vi "Init.vi"(8 "error in (no error)":errorcluster, 10 "Node Reg":refnum<k20>, 11 "Loop in":refnum<class "Loop.lvclass">) -> (0 "error out":errorcluster, 3 "Loop out":refnum<class "Loop.lvclass">)   [LabVIEW 2025, in "Loop.lvclass"]
uses:
  Loop.lvclass
  Controls/Shift Register.ctl
  Controls/Terminal.ctl
  Structure.lvclass
  <vilib>/xml/NI_XML.lvlib
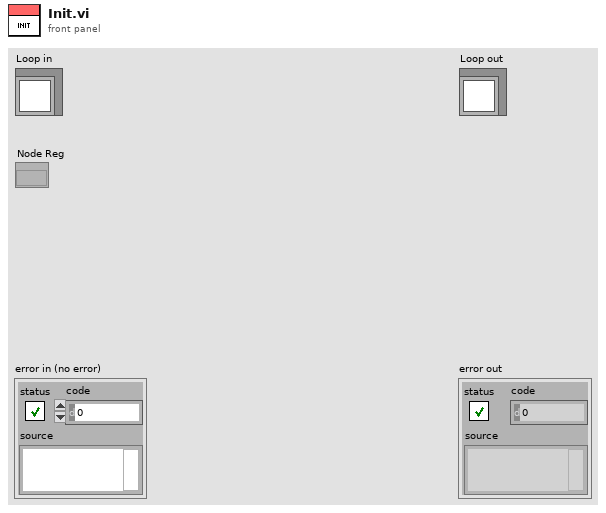
[diagram p1: front panel]
types:
  T1 = typedef "Shift Register.ctl" = cluster{"name":string, "LH Ext":T2, "LH Int":T2, "RH Int":T2, "RH Ext":T2, "Y pos":u32}
  T2 = typedef "Terminal.ctl" = cluster{"id":string, "name":string, "terminal":refnum<vi>}
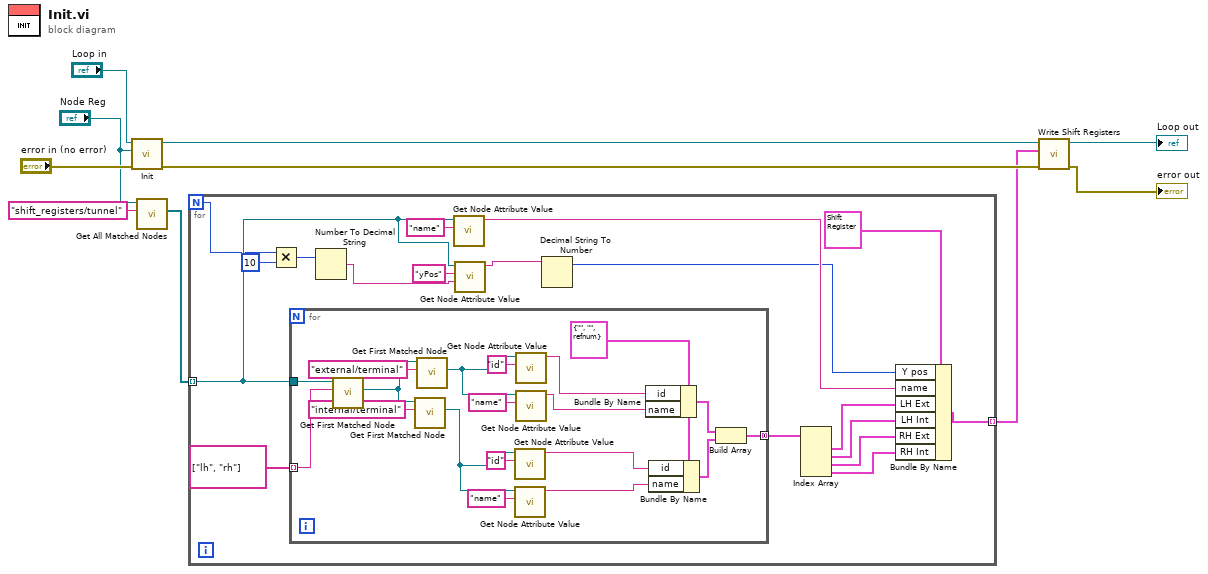
[diagram p0: block diagram]
diagram:
  n1 = call-parent "Init.vi"("error in (no error)"="error in (no error)", "Node Reg"="Node Reg", "Structure in"="Loop in") -> ("error out"=w8:errorcluster, "Structure out"=w7:refnum<class "Loop.lvclass">)  [unwired: 7 in]
  n2 = call <vilib>:"Get All Matched Nodes.vi"("XPath expression"="shift_registers/tunnel", "node in"="Node Reg") -> ("node result array"=w2:refnum<k20>[])  [unwired: 7 in, 2 out]
  n3 = for {
    N -> [w14]
    tunnel: w2 -> [w18] mode=indexing
    tunnel: [w19] -> w1 mode=indexing
    n4 = Multiply(x=w14, y=10) -> (x*y=w12:i32)
    n5 = for {
      tunnel: w18 -> [w47]
      tunnel: string[] ["lh", "rh"] -> [w46] mode=indexing
      tunnel: [w29] -> w27 mode=concatenating
      w34 = T2 {"id"="", "name"="", "terminal"=refnum} ("Terminal")
      n6 = call <vilib>:"Get First Matched Node.vi"("XPath expression"=w46, "node in"=w47) -> ("node result"=w45:refnum<k20>)  [unwired: 7 in, 2 out]
      n7 = call <vilib>:"Get First Matched Node.vi"("XPath expression"="internal/terminal", "node in"=w45) -> ("node result"=w37:refnum<k20>)  [unwired: 7 in, 2 out]
      n8 = call <vilib>:"Get First Matched Node.vi"("XPath expression"="external/terminal", "node in"=w45) -> ("node result"=w41:refnum<k20>)  [unwired: 7 in, 2 out]
      n9 = call "Get Node Attribute Value.vi"("Attribute Name"="id", "Refnum in"=w37) -> ("Value"=w33:string)  [unwired: 9 in]
      n10 = call "Get Node Attribute Value.vi"("Attribute Name"="name", "Refnum in"=w37) -> ("Value"=w32:string)  [unwired: 9 in]
      n11 = call "Get Node Attribute Value.vi"("Attribute Name"="id", "Refnum in"=w41) -> ("Value"=w36:string)  [unwired: 9 in]
      n12 = call "Get Node Attribute Value.vi"("Attribute Name"="name", "Refnum in"=w41) -> ("Value"=w35:string)  [unwired: 9 in]
      n13 = Bundle By Name(cluster=w34, "id"=w36, "name"=w35) -> (w31:T2)
      n14 = Bundle By Name(cluster=w34, "id"=w33, "name"=w32) -> (w30:T2)
      n15 = Build Array(w31, w30) -> (w29:T2[])
    }
    n16 = Number To Decimal String(number=w12) -> (decimal integer string=w11:string)  [unwired: 1 in]
    n17 = call "Get Node Attribute Value.vi"("Attribute Name"="name", "Refnum in"=w18) -> ("Value"=w24:string)  [unwired: 9 in]
    n18 = call "Get Node Attribute Value.vi"("Default Value"=w11, "Attribute Name"="yPos", "Refnum in"=w18) -> ("Value"=w16:string)  [unwired: 8 in]
    n19 = Decimal String To Number(string=w16) -> (offset past number=w15:i32)  [unwired: 2 in, 1 out]
    n20 = Index Array(array=w27) -> (element #1=w23:T2, element #2=w22:T2, element #3=w21:T2, element #4=w20:T2)  [unwired: 4 in]
    n21 = Bundle By Name(cluster=T1 {"name"="", "LH Ext"={"id"="", "name"="", "terminal"=refnum}, "LH Int"={"id"="", "name"="", "terminal"=refnum}, "RH Int"={"id"="", "name"="", "terminal"=refnum}, "RH Ext"={"id"="", "name"="", "terminal"=refnum}, "Y pos"=0} ("Shift Register"), "Y pos"=w15, "name"=w24, "LH Ext"=w23, "LH Int"=w22, "RH Ext"=w21, "RH Int"=w20) -> (w19:T1)
  }
  n22 = call-dynamic "Write Shift Registers.vi"("error in (no error)"=w8, "Shift Registers"=w1, "Loop in"=w7) -> ("error out"=→"error out":errorcluster, "Loop out"=→"Loop out":refnum<class "Loop.lvclass">)  [unwired: 7 in]
